vi "Process Measurement.vi"(0 "Waveform":waveform(dbl), 11 "error in":errorcluster) -> (4 "Test Values":T1, 15 "error out":errorcluster)   [LabVIEW 2023, in "AI.lvlib"]
uses:
  AI.lvlib
  Test Values.ctl
  <vilib>/measure/mascope.llb/Transition Measurements 1 chan.vi
  <vilib>/measure/mascope.llb/Amplitude and Levels 1 chan.vi
  <vilib>/measure/NI_MAPro.lvlib
panel:
  out "low state level":dbl format="%.2g"
  out "high state level":dbl format="%.2g"
  out "Rise time":dbl
  out "Fall time":dbl
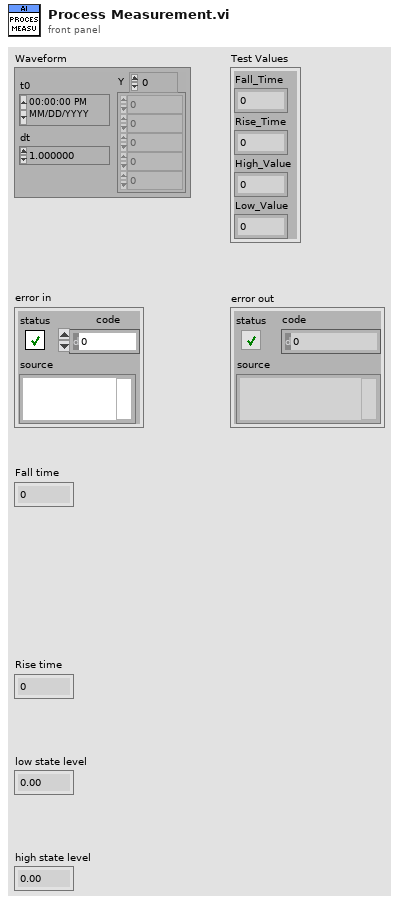
[diagram p1: front panel]
types:
  T1 = typedef "AI.lvlib/Test Values.ctl" = cluster{"Fall_Time":dbl, "Rise_Time":dbl, "High_Value":dbl, "Low_Value":dbl}
  T2 = cluster{"method":enum32{"histogram", "peak", "auto select"}, "histogram size":i32, "histogram method":enum16{"mode"}, "reserved":dbl}
  T3 = cluster{"high ref level":dbl, "mid ref level":dbl, "low ref level":dbl, "ref units":u16}
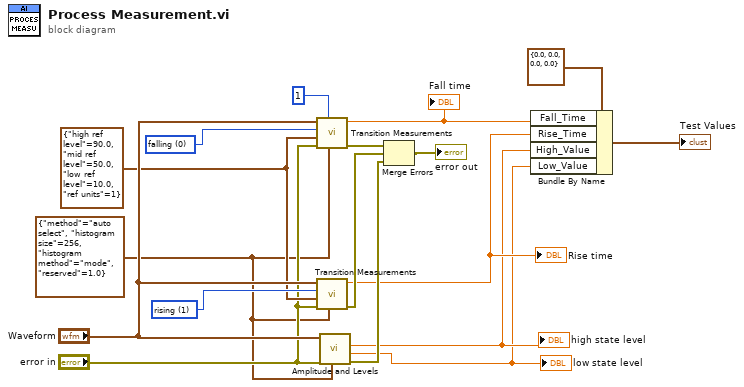
[diagram p0: block diagram]
diagram:
  w11 = T2 {"method"=enum."auto select", "histogram size"=256, "histogram method"=enum."mode", "reserved"=1.0} ("percent level settings")
  w14 = T3 {"high ref level"=90.0, "mid ref level"=50.0, "low ref level"=10.0, "ref units"=1} ("reference levels")
  w16 = u16 0 items=["falling", "rising"] ("polarity (rising)")
  w17 = u16 1 items=["falling", "rising"] ("polarity (rising)")
  n1 = call-poly <vilib>:"Transition Measurements.vi"("percent level settings"=w11, "edge number (1)"=1, "error in (no error)"="error in", "reference levels"=w14, "polarity (rising)"=w16, "signal in"="Waveform") -> ("error out"=w10:errorcluster, "transition duration"=w5:dbl)  [unwired: 4 out]
  "Fall time" <- w5
  n2 = call-poly <vilib>:"Transition Measurements.vi"("percent level settings"=w11, "error in (no error)"="error in", "reference levels"=w14, "polarity (rising)"=w17, "signal in"="Waveform") -> ("error out"=w9:errorcluster, "transition duration"=w4:dbl)  [unwired: 1 in, 4 out]
  "Rise time" <- w4
  n3 = call-poly <vilib>:"Amplitude and Levels.vi"("state settings"=w11, "error in (no error)"="error in", "signal in"="Waveform") -> ("error out"=w8:errorcluster, "low state level"=w2:dbl, "high state level"=w3:dbl)  [unwired: 5 in, 1 out]
  "high state level" <- w3
  "low state level" <- w2
  n4 = Merge Errors(w10, w9, w8) -> (→"error out":errorcluster)
  n5 = Bundle By Name(cluster=T1 {"Fall_Time"=0.0, "Rise_Time"=0.0, "High_Value"=0.0, "Low_Value"=0.0}, "Fall_Time"=w5, "Rise_Time"=w4, "High_Value"=w3, "Low_Value"=w2) -> (→"Test Values":T1)
